vi "Multi-nRF24-BME280-Logger-v1.1.0.vi"() -> ()   [LabVIEW 2018]
uses:
  Program Files (x86)/National Instruments/LabVIEW 2018/examples/Instrument IO/Serial/support/Serial - XON-XOFF Characters.ctl
  Program Files (x86)/National Instruments/LabVIEW 2018/examples/Instrument IO/Serial/support/Serial - ASCII Characters.ctl
  Program Files (x86)/National Instruments/LabVIEW 2018/examples/Instrument IO/Serial/support/Serial - Settings.ctl
  <vilib>/Instr/_visa.llb/VISA Configure Serial Port (Instr).vi
panel:
  out "Logs Paths":path[](array[path])
  out "Humidity 2":dbl(knob) scale=0.0..100.0
  out "Temperature 2":dbl(slide) scale=0.0..100.0
  out "Temperature 1":dbl(slide) scale=0.0..100.0
  out "Humidity 1":dbl(knob) scale=0.0..100.0
  in  "Start Button":bool
  out "Log String":string
  out "error out":errorcluster
  in  "VISA resource name":refnum<visa-resource-name>="COM1"
  out "Response":string
  in  "Stop":bool
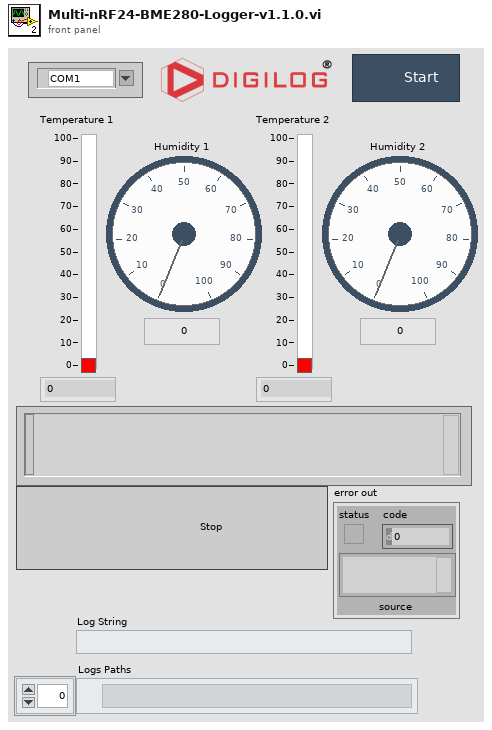
[diagram p1: front panel]
types:
  T1 = typedef "Serial - Settings.ctl" = cluster{"baud rate":u32, "data bits":u16, "parity":enum16{"None", "Odd", "Even", "Mark", "Space"}, "stop bits":u16, "flow control":u16}
  T2 = typedef "Serial - XON-XOFF Characters.ctl" = cluster{"XON":T3, "XOFF":T3}
  T3 = typedef "Serial - ASCII Characters.ctl" = enum16{"NUL", "SOH", "STX", "ETX", "EOT", "ENQ", "ACK", "BEL", "BS", "HT", "LF", "VT", "FF", "CR", "SO", "SI", "DLE", "DC1", "DC2", "DC3", "DC4", "NAK", "SYN", "ETB", "CAN", "EM", "SUB", "ESC", "FS", "GS", "RS", "US", "SP", "!", "\"", "#", "$", "%", "&", "'", "(", ")", "*", "+", ",", "- (-)", ".", "/", "0", "1", "2", "3", "4", "5", "6", "7", "8", "9", ":", ";", "<", "=", ">", "?", "@", "A", "B", "C", "D", "E", "F", "G", "H", "I", "J", "K", "L", "M", "N", "O", "P", "Q", "R", "S", "T", "U", "V", "W", "X", "Y", "Z", "[", "\\", "]", "^", "_", "`", "a", "b", "c", "d", "e", "f", "g", "h", "i", "j", "k", "l", "m", "n", "o", "p", "q", "r", "s", "t", "u", "v", "w", "x", "y", "z", "{", "|", "}", "~"}
  T4 = enum16{"open", "replace", "create", "open or create", "replace or create", "replace or create with confirmation"}
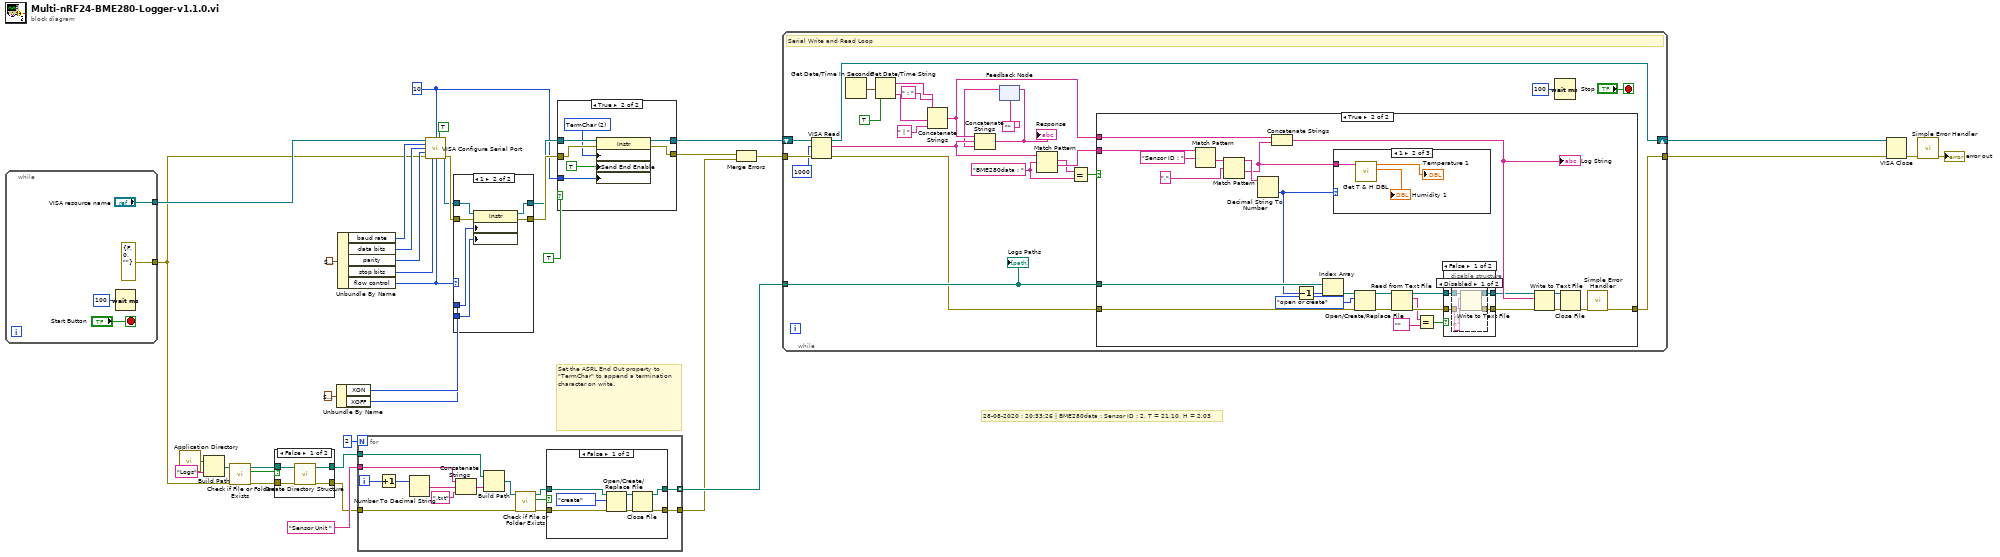
[diagram p0: block diagram]
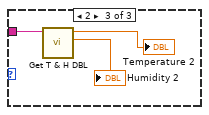
[diagram p6: hidden frame]
diagram:
  w8 = u8 10 ("Termination Character")
  # "28-08-2020 : 20:33:26 | BME280data : Sensor ID : 2, T = 21.10, H = 2.03"
  # "Set the ASRL End Out property to \"TermChar\" to append a termination character on write."
  n1 = while {
    tunnel: ["VISA resource name"] -> w28
    tunnel: [errorcluster {"status"=FALSE, "code"=0, "source"=""} ("error in (no error)")] -> w6
    stop <- "Start Button" stop-if-true
    n2 = Wait (ms)(milliseconds to wait=u32 100) -> ()  [unwired: 1 out]
  }
  n3 = call <vilib>:"Application Directory.vi"() -> ("Application Directory"=w29:path)
  n4 = Build Path(base path=w29, name or relative path="Logs") -> (appended path=w36:path)
  n5 = call <vilib>:"Check if File or Folder Exists.vi"("error in (no error)"=w6, "path"=w36) -> ("error out"=w32:errorcluster, "file or folder exists?"=w34:bool, "dup path"=w33:path)  [unwired: 7 in]
  n6 = case shown="False" w34 {
    tunnel: w33 -> [w45 w47]
    tunnel: w32 -> [w44 w46]
    tunnel: [w43 w47] -> w31
    tunnel: [w42 w46] -> w30
    frame False {
      n7 = call "Create Directory Structure.vi"("error in(no error)"=w44, "Dir Path In"=w45) -> ("error out"=w42:errorcluster, "Dir Path Out"=w43:path)  [unwired: 8 in]
    }
    frame True {
    }
  }
  n8 = Unbundle By Name(T2 {"XON"=enum."DC1", "XOFF"=enum."DC3"} ("XON/XOFF Characters")) -> ("XON"=w14:T3, "XOFF"=w13:T3)
  n9 = Unbundle By Name(T1 {"baud rate"=115200, "data bits"=8, "parity"=enum."None", "stop bits"=10, "flow control"=0} ("Serial Settings")) -> ("baud rate"=w21:u32, "data bits"=w22:u16, "parity"=w23:enum16{"None", "Odd", "Even", "Mark", "Space"}, "stop bits"=w24:u16, "flow control"=w15:u16)
  n10 = for {
    N: 2 -> [_]
    tunnel: "Sensor Unit " ("name or relative path") -> [w59]
    tunnel: w31 -> [w55]
    tunnel: w30 -> [w53]
    tunnel: [w49] -> w5 mode=indexing
    tunnel: [w48] -> w4
    i -> [w61]
    n11 = Increment(x=w61) -> (x+1=w60:i32)
    n12 = Number To Decimal String(number=w60) -> (decimal integer string=w58:string)  [unwired: 1 in]
    n13 = Concatenate Strings(w59, w58, ".txt" ("string")) -> (w56:string)
    n14 = Build Path(base path=w55, name or relative path=w56) -> (appended path=w54:path)
    n15 = call <vilib>:"Check if File or Folder Exists.vi"("error in (no error)"=w53, "path"=w54) -> ("error out"=w50:errorcluster, "file or folder exists?"=w52:bool, "dup path"=w51:path)  [unwired: 7 in]
    n16 = case shown="False" w52 {
      tunnel: w51 -> [w66 w70]
      tunnel: w50 -> [w67 w69]
      tunnel: [w64 w70] -> w49
      tunnel: [w62 w69] -> w48
      frame False {
        n17 = Open/Create/Replace File(file path (use dialog)=w66, error in=w67, operation (0:open)=T4."create") -> (refnum out=w65:refnum<file>, error out=w63:errorcluster)  [unwired: 3 in, 1 out]
        n18 = Close File(refnum=w65, error in=w63) -> (path=w64:path, error out=w62:errorcluster)
      }
      frame True {
      }
    }
  }
  n19 = call-poly "VISA Configure Serial Port"("VISA resource name"=w28, "termination char\n(0xA = '\\n' = LF)"=w8, "Enable Termination\nChar (T)"=TRUE ("End Read on Termination Character?"), "baud rate (9600)"=w21, "data bits (8)"=w22, "parity (0:none)"=w23, "error in (no error)"=w6, "stop bits (10: 1 bit)"=w24, "flow control (0:none)"=w15) -> ("VISA resource name out"=w25:refnum<visa-resource-name>, "error out"=w26:errorcluster)  [unwired: 1 in, 4 out]
  n20 = case shown="1" w15 {
    tunnel: [w71 w78] -> w12
    tunnel: [w72 w77] -> w11
    tunnel: w26 -> [w71 w76]
    tunnel: w25 -> [w72 w75]
    tunnel: w14 -> [_ w74]
    tunnel: w13 -> [_ w73]
    frame Default {
    }
    frame 1 {
      n21 = property class="Instr"(reference=w75, error in=w76, "Serial Settings:Flow Control XON Character"=w74, "Serial Settings:Flow Control XOFF Character"=w73) -> (reference out=w77:refnum<visa-resource-name>, error out=w78:errorcluster)
    }
  }
  n22 = case shown="True" TRUE ("End Write on Termination Character?") {
    tunnel: w11 -> [w79 w87]
    tunnel: w12 -> [w80 w86]
    tunnel: [w79 w85] -> w10
    tunnel: [w80 w84] -> w3
    tunnel: w8 -> [_ w82]
    frame False {
    }
    frame True {
      w83 = u16 2 items=["None", "LastBit", "TermChar", "Break"] ("Serial Settings:Serial End Mode for Writes")
      n23 = property class="Instr"(reference=w87, error in=w86, "Serial Settings:End Mode for Writes"=w83, "Message Based Settings:Send End Enable"=TRUE, "Message Based Settings:Termination Character"=w82) -> (reference out=w85:refnum<visa-resource-name>, error out=w84:errorcluster)
    }
  }
  n24 = Merge Errors(w3, w4) -> (w2:errorcluster)
  n25 = while {
    shift-right: [w106] -> w16
    shift-left: w10 -> [w111]
    tunnel: w2 -> [w110]
    tunnel: [w89] -> w17
    tunnel: w5 -> [w91]
    stop <- "Stop" stop-if-true
    w93 = "BME280data : "
    # "Serial Write and Read Loop"
    n26 = VISA Read(VISA resource name=w111, byte count=u32 1000 ("Read Count"), error in (no error)=w110) -> (VISA resource name out=w106:refnum<visa-resource-name>, read buffer=w92:string, error out=w90:errorcluster)  [unwired: 1 out]
    n27 = Get Date/Time In Seconds() -> (seconds since 1Jan1904=w102:timestamp)
    n28 = Get Date/Time String(seconds (now)=w102, want seconds? (F)=TRUE) -> (date string=w103:string, time string=w101:string)  [unwired: 1 in]
    n29 = Concatenate Strings(w103, " : " ("string"), w101, " | " ("string")) -> (w104:string)
    n30 = feedback #1("") -> (w88:string)
    n31 = Concatenate Strings(w104, w92, w88) -> (w105:string)
    "Response" <- w105
    n32 = feedback-in #1(w105) -> ()
    n33 = Match Pattern(string=w92, regular expression=w93) -> (match substring=w98:string, after substring=w100:string)  [unwired: 1 in, 2 out]
    n34 = Equal?(x=w98, y=w93) -> (x = y?=w99:bool)
    n35 = case shown="True" w99 {
      tunnel: w100 -> [_ w139]
      tunnel: w104 -> [_ w132]
      tunnel: w91 -> [_ w134]
      tunnel: w90 -> [w112 w125]
      tunnel: [w112 w124] -> w89
      frame False {
      }
      frame True {
        n36 = Match Pattern(string=w139, regular expression="Sensor ID : ") -> (after substring=w137:string)  [unwired: 1 in, 3 out]
        n37 = Match Pattern(string=w137, regular expression=",") -> (before substring=w135:string, after substring=w114:string)  [unwired: 1 in, 2 out]
        n38 = Decimal String To Number(string=w135) -> (number=w113:i32)  [unwired: 2 in, 1 out]
        n39 = Concatenate Strings(w132, w114) -> (w126:string)
        "Log String" <- w126
        n40 = Decrement(x=w113) -> (x-1=w133:i32)
        n41 = Index Array(array=w134, index=w133) -> (element=w127:path)
        n42 = case shown="1" w113 {
          tunnel: w114 -> [_ w142 w145]
          frame 0, Default {
          }
          frame 1 {
            n43 = call "Get T & H DBL.vi"("String Input"=w142) -> ("H DBL"=→"Humidity 1":dbl, "T DBL"=→"Temperature 1":dbl)  [unwired: 9 in]
          }
          frame 2 {
            n44 = call "Get T & H DBL.vi"("String Input"=w145) -> ("H DBL"=→"Humidity 2":dbl, "T DBL"=→"Temperature 2":dbl)  [unwired: 9 in]
          }
        }
        n45 = Open/Create/Replace File(file path (use dialog)=w127, error in=w125, operation (0:open)=T4."open or create") -> (refnum out=w118:refnum<file>, error out=w117:errorcluster)  [unwired: 3 in, 1 out]
        n46 = Read from Text File(file (use dialog)=w118, error in=w117) -> (refnum out=w123:refnum<file>, text=w121:string, error out=w122:errorcluster)  [unwired: 2 in, 1 out]
        n47 = Equal?(x=w121, y="" ("string")) -> (x = y?=w120:bool)
        n48 = case shown="False" w120 {
          tunnel: w123 -> [w149 w158]
          tunnel: [w148 w158] -> w116
          tunnel: w122 -> [w147 w157]
          tunnel: [w146 w157] -> w115
          frame False {
            n49 = disable-structure shown="Disabled" {
              disable-tunnel: w149 -> [w153 w156]
              disable-tunnel: [w152 w156] -> w148
              disable-tunnel: w147 -> [w151 w155]
              disable-tunnel: [w150 w155] -> w146
              frame Disabled {
                n50 = Write to Text File(file (use dialog)=w153, text="\n", error in=w151) -> (refnum out=w152:refnum<file>, error out=w150:errorcluster)  [unwired: 1 in, 1 out]
              }
              frame Enabled {
              }
            }
          }
          frame True {
          }
        }
        n51 = Write to Text File(file (use dialog)=w116, text=w126, error in=w115) -> (refnum out=w130:refnum<file>, error out=w131:errorcluster)  [unwired: 1 in, 1 out]
        n52 = Close File(refnum=w130, error in=w131) -> (error out=w128:errorcluster)  [unwired: 1 out]
        n53 = call <vilib>:"Simple Error Handler.vi"("error in (no error)"=w128) -> ("error out"=w124:errorcluster)  [unwired: 4 in, 4 out]
      }
    }
    n54 = Wait (ms)(milliseconds to wait=u32 100) -> ()  [unwired: 1 out]
    "Logs Paths" <- w91
  }
  n55 = VISA Close(VISA resource name=w16, error in (no error)=w17) -> (error out=w18:errorcluster)
  n56 = call <vilib>:"Simple Error Handler.vi"("error in (no error)"=w18) -> ("error out"=→"error out":errorcluster)  [unwired: 1 in, 7 out]
